vi "RequestTemplate.vi"(6 "timeout in ms (-1)":i32=-1, 8 "error in (no error)":errorcluster, 11 "module in":refnum<class>) -> (0 "error out":errorcluster, 3 "module out":refnum<class>, 4 "timed out?":bool)   [LabVIEW 2024, in "AddNewEvent.lvlib"]
uses:
  Event/AddNewEvent.lvlib
  JQMHCore/Module/RQMHModule.lvclass
  JQMHCore/Module/Reply.ctl
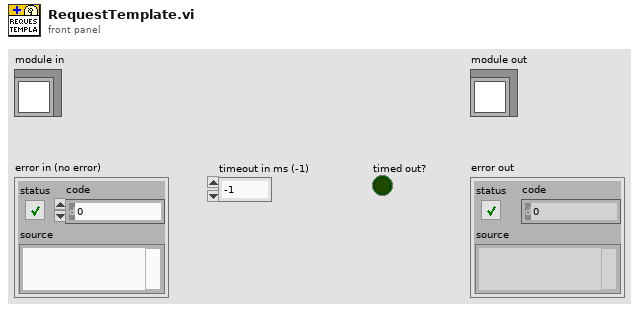
[diagram p1: front panel]
types:
  T1 = typedef "RQMHModule.lvclass/Reply.ctl" = cluster{"Expects Reply":bool, "Reply":refnum<notifier>}
  T2 = cluster{"RQMH_REPLYARGS":cluster{}, "error in (no error)":errorcluster}
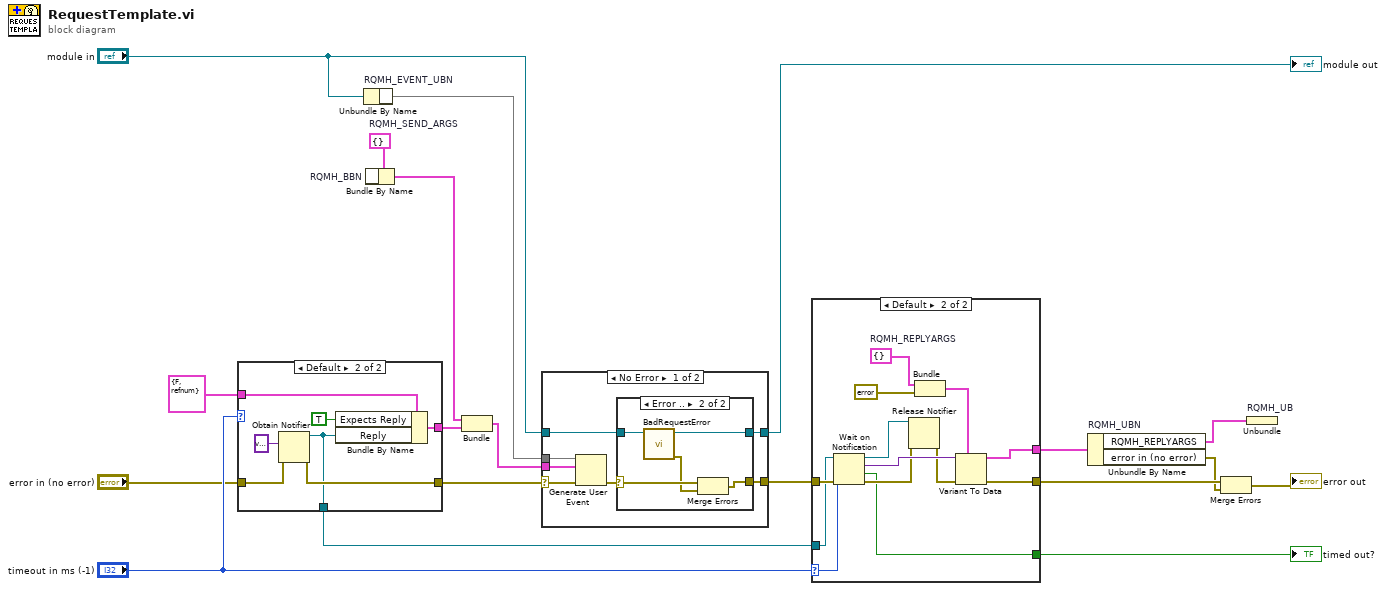
[diagram p0: block diagram]
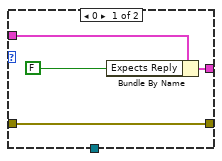
[diagram p4: hidden frame]
diagram:
  w9 = cluster{} {}  # RQMH_SEND_ARGS
  n1 = case shown="Default" "timeout in ms (-1)" {
    tunnel: [w22 w29] -> w19
    tunnel: "error in (no error)" -> [w20 w28]
    tunnel: [w20 w27] -> w17
    tunnel: [_ w26] -> w15
    tunnel: T1 {"Expects Reply"=FALSE, "Reply"=refnum} ("Reply") -> [w23 w25]
    frame 0 {
      n2 = Bundle By Name(cluster=w23, "Expects Reply"=FALSE) -> (w22:T1)
    }
    frame Default {
      n3 = Obtain Notifier(notification data type=variant, error in (no error)=w28) -> (notifier out=w26:refnum<notifier>, error out=w27:errorcluster)  [unwired: 2 in, 1 out]
      n4 = Bundle By Name(cluster=w25, "Expects Reply"=TRUE, "Reply"=w26) -> (w29:T1)
    }
  }
  n5 = Unbundle By Name "RQMH_EVENT_UBN"("module in") -> (w7)
  n6 = Bundle By Name "RQMH_BBN"(cluster=w9) -> (w6:cluster{})  [unwired: 1 in]
  n7 = Bundle("RQMH_SEND_ARGS"=w6, "Reply"=w19) -> (w18:cluster{"RQMH_SEND_ARGS":cluster{}, "Reply":T1})  [unwired: 1 in]
  n8 = case shown="No Error" w17 {
    selector: w17 -> [w34 w45]
    tunnel: w18 -> [w37 _]
    tunnel: w7 -> [w36 _]
    tunnel: [w33 w45] -> w16
    tunnel: "module in" -> [w32 w46]
    tunnel: [w31 w46] -> w10
    frame No Error {
      n9 = Generate User Event(user event=w36, event data cluster=w37, error in=w34) -> (error out=w35:errorcluster)  [unwired: 1 in, 1 out]
      n10 = case shown="Error .." w35 {
        selector: w35 -> [w38 w44]
        tunnel: [w38 w43] -> w33
        tunnel: w32 -> [w39 w42]
        tunnel: [w39 w41] -> w31
        frame No Error {
        }
        frame Error {
          n11 = call "BadRequestError.vi"("JQMHModule in"=w42) -> ("error out"=w40:errorcluster, "JQMHModule out"=w41:refnum<class "RQMHModule.lvclass">)  [unwired: 9 in]
          n12 = Merge Errors(w44, w40) -> (w43:errorcluster)
        }
      }
    }
    frame Error {
    }
  }
  "module out" <- w10
  n13 = case shown="Default" "timeout in ms (-1)" {
    selector: "timeout in ms (-1)" -> [_ w51]
    tunnel: w16 -> [w47 w60]
    tunnel: w15 -> [_ w59]
    tunnel: [_ w52] -> w14
    tunnel: [w47 w49] -> w5
    tunnel: [_ w48] -> w4
    frame 0 {
    }
    frame Default {
      w50 = cluster{} {}  # RQMH_REPLYARGS
      n14 = Wait on Notification(notifier=w59, timeout in ms (-1)=w51, error in (no error)=w60) -> (notifier out=w55:refnum<notifier>, notification=w56:variant, timed out?=w52:bool, error out=w54:errorcluster)  [unwired: 1 in]
      n15 = Release Notifier(notifier=w55, error in (no error)=w54) -> (error out=w53:errorcluster)  [unwired: 1 in, 2 out]
      n16 = Bundle("RQMH_REPLYARGS"=w50, "error in (no error)"=errorcluster {"status"=FALSE, "code"=0, "source"=""}) -> (w58:T2)  [unwired: 1 in]
      n17 = Variant To Data(error in=w53, type=w58, Variant=w56) -> (data=w48:T2, error out=w49:errorcluster)
    }
  }
  "timed out?" <- w14
  n18 = Unbundle By Name "RQMH_UBN"(w4) -> ("RQMH_REPLYARGS"=w1:cluster{}, "error in (no error)"=w2:errorcluster)
  n19 = Merge Errors(w5, w2) -> (→"error out":errorcluster)
  n20 = Unbundle "RQMH_UB"(w1) -> ()  [unwired: 1 out]
